vi "Serialize - JSON.vi"(8 "error in":errorcluster, 11 "Vaisala Data in":refnum<class "Vaisala Data.lvclass">) -> (0 "error out":errorcluster, 2 "Serialized JSON":string, 3 "Vaisala Data out":refnum<class "Vaisala Data.lvclass">)   [LabVIEW 2014, in "Vaisala Library.lvlib" / "Vaisala Data.lvclass"]
uses:
  Vaisala Data.lvclass
  reusable/Data/Data.lvclass/Data.ctl
  Vaisala Data.lvclass/Vaisala Data.ctl
  reusable/Data/Read Data ID.vi
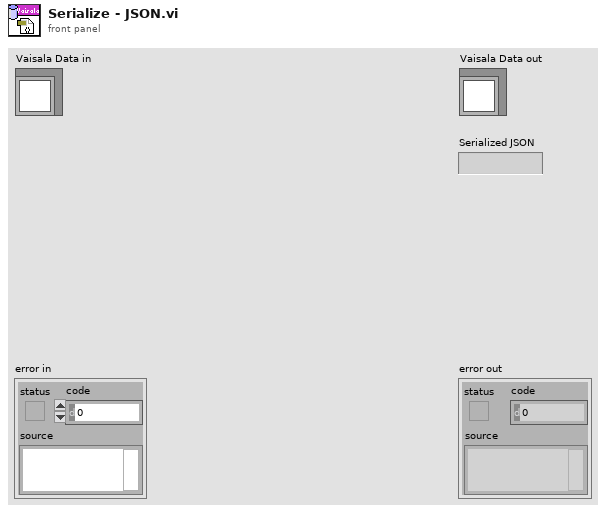
[diagram p1: front panel]
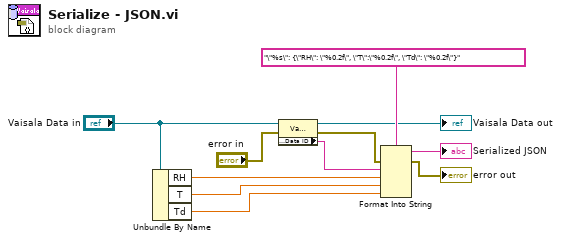
[diagram p0: block diagram]
diagram:
  n1 = Unbundle By Name("Vaisala Data in") -> ("RH"=w3:dbl, "T"=w2:dbl, "Td"=w1:dbl)
  n2 = property class="Vaisala Data"(reference="Vaisala Data in", error in="error in") -> (reference out=→"Vaisala Data out":refnum<class "Vaisala Data.lvclass">, error out=w6:errorcluster, "Accessors:Data ID"=w8:string)
  n3 = Format Into String(format string="\"%s\": {\"RH\": \"%0.2f\", \"T\":\"%0.2f\", \"Td\": \"%0.2f\"}", error in=w6, w8, w3, w2, w1) -> (resulting string=→"Serialized JSON":string, error out=→"error out":errorcluster)  [unwired: 1 in]
